vi "Go To Target_recreate.vi"(4 "Safe Distance (Inches)":i32, 5 "Sonar Distance (Inches)":i32, 6 "Center Tolerance":i32, 7 "Distance We Want":i32, 8 "Rotation Speed":dbl, 9 "Foward Speed":dbl, 10 "Objects Position":i32, 11 "Distance":i32) -> ()   [LabVIEW 2014]
uses:
  <vilib>/Rock Robotics/WPI/RobotDrive/WPI_RobotDriveGetSetRefNum.vi
  <vilib>/Rock Robotics/WPI/RobotDrive/WPI_RobotDriveMecanumDrive_Cartesian.vi
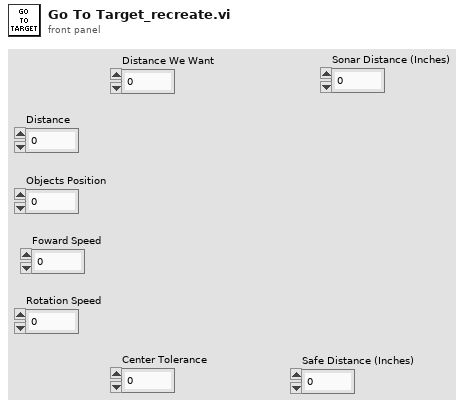
[diagram p1: front panel]
types:
  T1 = typedef "WPI_RobotDriveDevRef.ctl" = cluster{"DevStatus":errorcluster, "Motors[]":T2[], "Square Inputs":bool, "Max Output":dbl}
  T2 = typedef "WPI_MotorControlDeviceRef.ctl" = cluster{"DeviceStatus":errorcluster, "Type":T3, "PWM":cluster{"Controller":T4, "PWM Channel":T5, "DeadBand":T6}, "CAN":cluster{"Device Number":u8, "Control Mode":T7, "Semaphore":T8, "Max Vout":dbl, "TalonSRX Control Mode":T9}, "Invert":bool, "TransformRef":T10, "InvTransformRef":T10}
  T3 = typedef "WPI_MotorControlType.ctl" = enum16{"PWM", "CAN", "CANTalonSRX"}
  T4 = typedef "FPGA_TypedefDigitalModule.ctl" = enum16{"Controller 1"}
  T5 = typedef "FPGA_DIOPWMChannel.ctl" = enum8{"PWM 0", "PWM 1", "PWM 2", "PWM 3", "PWM 4", "PWM 5", "PWM 6", "PWM 7", "PWM 8", "PWM 9", "PWM MXP 0", "PWM MXP 1", "PWM MXP 2", "PWM MXP 3", "PWM MXP 4", "PWM MXP 5", "PWM MXP 6", "PWM MXP 7", "PWM MXP 8", "PWM MXP 9", "Invalid"}
  T6 = typedef "WPI_PWMDeadband.ctl" = cluster{"Name":string, "maxPositivePwm":i32, "minPositivePwm":i32, "centerPwm":i32, "maxNegativePwm":i32, "minNegativePwm":i32, "angularRange":u16}
  T7 = typedef "WPI_CANJaguar_ControlMode.ctl" = enum8{"Percent VBus", "Current", "Speed", "Position", "Voltage"}
  T8 = typedef "Semaphore RefNum" = refnum<k1>
  T9 = typedef "WPI_CANTalonSRX_APIControlMode.ctl" = enum8{"Percent VBus", "Speed", "Position", "Slave", "Unchanged / Invalid"}
  T10 = typedef "WPI_PWMTransform_ConPane.ctl" = refnum<vi>
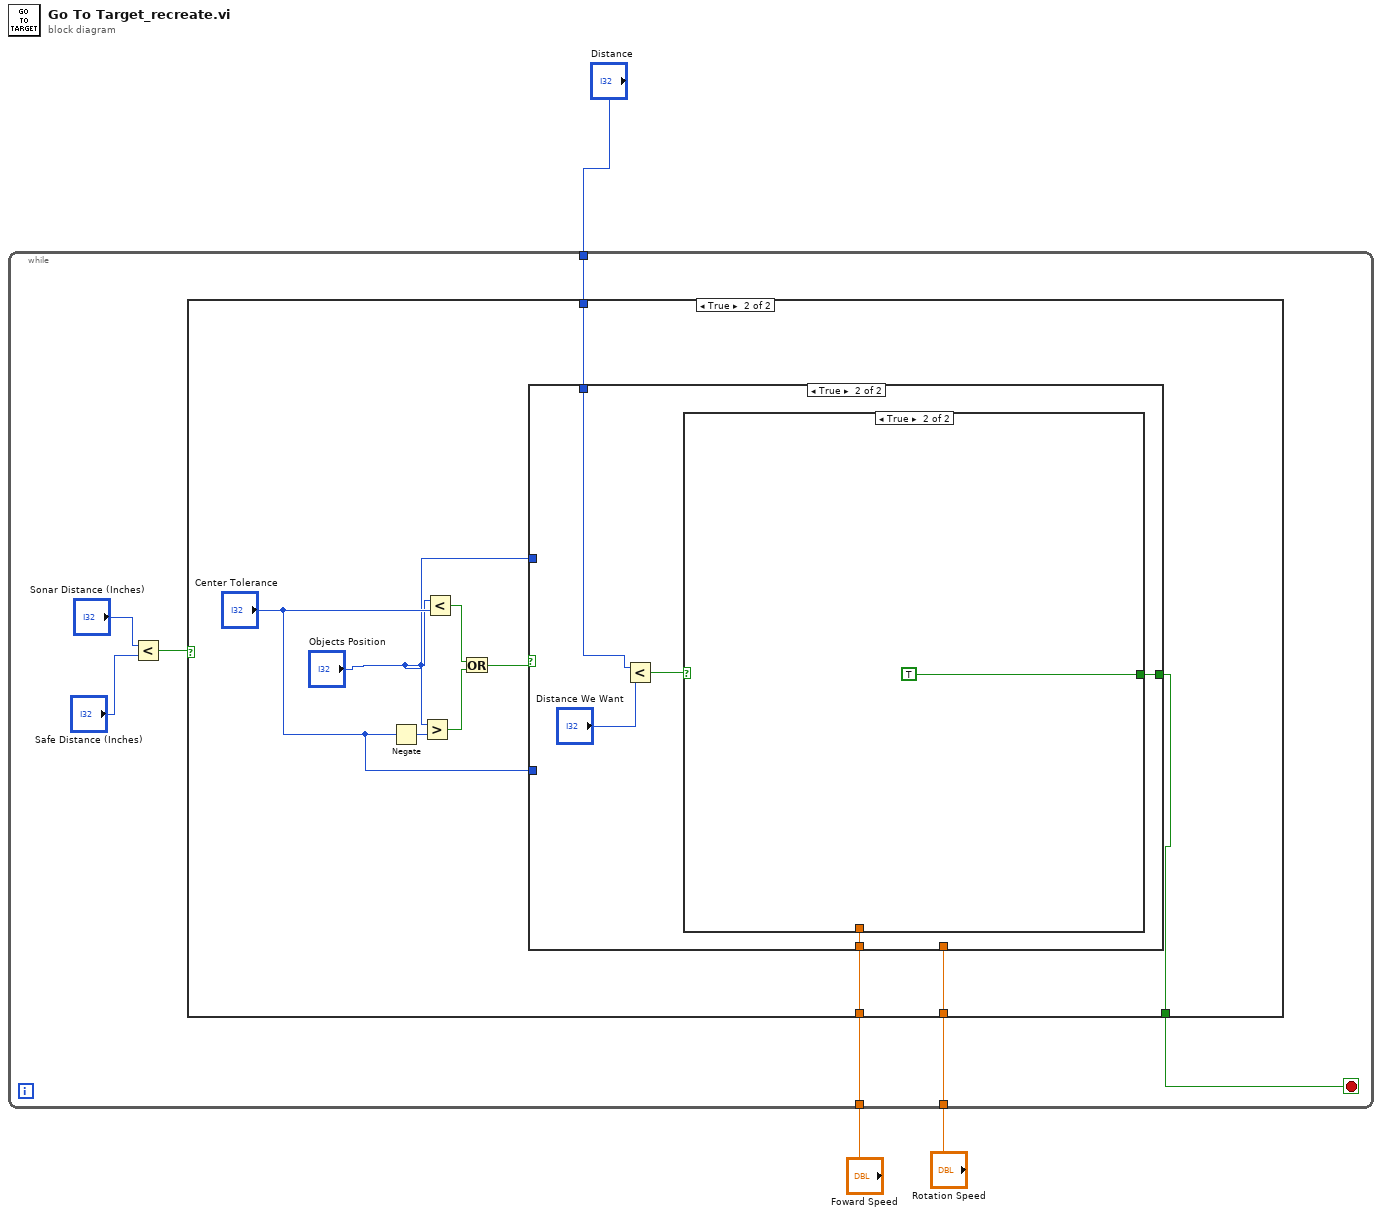
[diagram p0: block diagram]
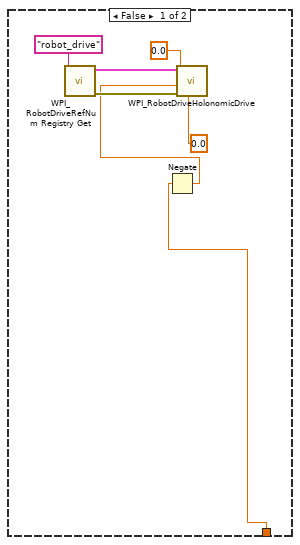
[diagram p2: hidden frame]
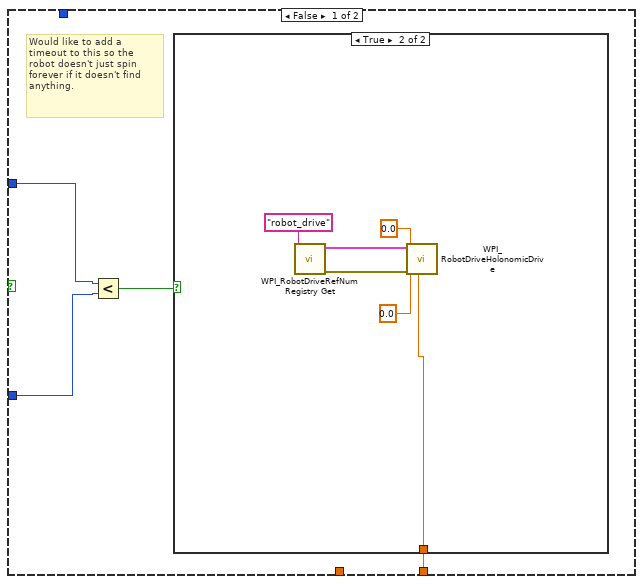
[diagram p3: hidden frame]
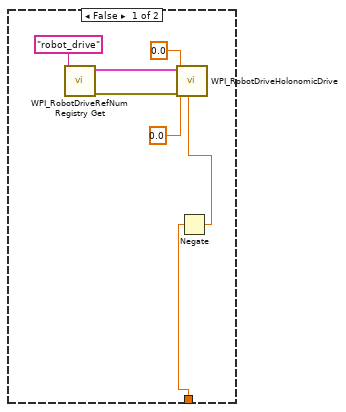
[diagram p4: hidden frame]
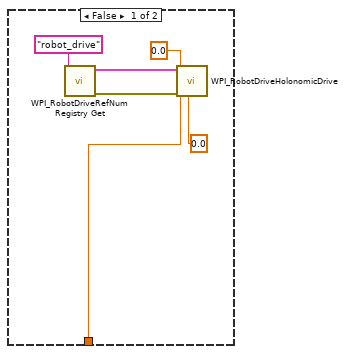
[diagram p5: hidden frame]
diagram:
  n1 = while {
    tunnel: "Rotation Speed" -> [w9]
    tunnel: "Foward Speed" -> [w8]
    tunnel: "Distance" -> [w7]
    stop <- w10 stop-if-true
    n2 = Less?(x="Sonar Distance (Inches)", y="Safe Distance (Inches)") -> (x < y?=w6:bool)
    n3 = case shown="True" w6 {
      tunnel: [_ w23] -> w10
      tunnel: w9 -> [_ w21]
      tunnel: w8 -> [w11 w20]
      tunnel: w7 -> [_ w18]
      frame False {
        n4 = call <vilib>:"WPI_RobotDriveRefNum Registry Get.vi"("refnum name"="robot_drive") -> ("error out"=w16:errorcluster, "RobotDriveDevRef"=w17:T1)  [unwired: 9 in]
        n5 = Negate(x=w11) -> (-x=w12:dbl)
        n6 = call-poly <vilib>:"WPI_RobotDriveHolonomicDrive.vi"("Rotation"=0.0, "error in (no error)"=w16, "Y"=w12, "X"=0.0, "RobotDriveDevRef"=w17) -> ()  [unwired: 4 in, 3 out]
      }
      frame True {
        n7 = Negate(x="Center Tolerance") -> (-x=w27:i32)
        n8 = Greater?(x="Objects Position", y=w27) -> (0:w25:bool)
        n9 = Less?(x="Objects Position", y="Center Tolerance") -> (x < y?=w26:bool)
        n10 = Or(x=w26, y=w25) -> (x .or. y?=w24:bool)
        n11 = case shown="True" w24 {
          tunnel: [_ w47] -> w23
          tunnel: "Objects Position" -> [w31 _]
          tunnel: "Center Tolerance" -> [w30 _]
          tunnel: w21 -> [w28 _]
          tunnel: w20 -> [_ w46]
          tunnel: w18 -> [_ w45]
          frame False {
            # "Would like to add a timeout to this so the robot doesn't just spin forever if it doesn't find anything."
            n12 = Less?(x=w31, y=w30) -> (x < y?=w29:bool)
            n13 = case shown="True" w29 {
              tunnel: w28 -> [w33 w39]
              frame False {
                n14 = call <vilib>:"WPI_RobotDriveRefNum Registry Get.vi"("refnum name"="robot_drive") -> ("error out"=w37:errorcluster, "RobotDriveDevRef"=w38:T1)  [unwired: 9 in]
                n15 = Negate(x=w33) -> (-x=w32:dbl)
                n16 = call-poly <vilib>:"WPI_RobotDriveHolonomicDrive.vi"("Rotation"=w32, "error in (no error)"=w37, "Y"=0.0, "X"=0.0, "RobotDriveDevRef"=w38) -> ()  [unwired: 4 in, 3 out]
              }
              frame True {
                n17 = call <vilib>:"WPI_RobotDriveRefNum Registry Get.vi"("refnum name"="robot_drive") -> ("error out"=w43:errorcluster, "RobotDriveDevRef"=w44:T1)  [unwired: 9 in]
                n18 = call-poly <vilib>:"WPI_RobotDriveHolonomicDrive.vi"("Rotation"=w39, "error in (no error)"=w43, "Y"=0.0, "X"=0.0, "RobotDriveDevRef"=w44) -> ()  [unwired: 4 in, 3 out]
              }
            }
          }
          frame True {
            n19 = Less?(x=w45, y="Distance We Want") -> (x < y?=w49:bool)
            n20 = case shown="True" w49 {
              tunnel: [_ TRUE] -> w47
              tunnel: w46 -> [w50 _]
              frame False {
                n21 = call <vilib>:"WPI_RobotDriveRefNum Registry Get.vi"("refnum name"="robot_drive") -> ("error out"=w54:errorcluster, "RobotDriveDevRef"=w55:T1)  [unwired: 9 in]
                n22 = call-poly <vilib>:"WPI_RobotDriveHolonomicDrive.vi"("Rotation"=0.0, "error in (no error)"=w54, "Y"=w50, "X"=0.0, "RobotDriveDevRef"=w55) -> ()  [unwired: 4 in, 3 out]
              }
              frame True {
              }
            }
          }
        }
      }
    }
  }
